vi "SVL Crest Factor (resampled) (1 Ch).vi"(6 "restart averaging (F)":bool, 8 "error in (no error)":errorcluster, 10 "even-angle channel info":T1={"channel name"="", "description"="", " channel info"={"sensor sensitivity"=1000.0, "engineering units"=1, "dB reference"=1.0, "custom label"="EU", "weighting filter"=0, "pregain"=0.0}} {"channel info"."pregain" format="%.2f"; "channel info"."weighting filter" items=["Linear", "A-weighting", "B-weighting", "C-weighting", "ITU-R 468-4", "Dolby", "CCITT", "C-message", "Wb", "Wc", "Wd", "We", "Wf", "Wh", "Wj", "Wk", "Wm", "AES17 20 kHz lowpass", "AES17 40 kHz lowpass", "AES17 20 kHz highpass", "AES17 40 kHz highpass"]; "channel info"."dB reference" format="%^.1e"; "channel info"."engineering units" items=["custom..."=0, "V"=1, "A"=21, "C"=30, "pC"=31, "s"=32, "-"=29, "Pa"=2, "N"=20, "g"=3, "m/s^2"=4, "m/s"=5, "m"=6, "mm/s"=12, "mm"=13, "micron/s"=14, "micron"=15, "in/s^2"=7, "in/s"=8, "in"=9, "mil/s"=10, "mil"=11, "rad/s^2"=16, "rad/s"=17, "rad"=18, "deg/s^2"=26, "deg/s"=27, "deg"=28, "RPM"=22, "cycle/s^2"=23, "Hz"=24, "cycle"=25, "strain"=19]; "channel info"."sensor sensitivity" format="%#_5f"}, 11 "even-angle signal [EU]":T5 {"even-angle signal" format="%.2f"; "dr" format="%.2f"; "r0" format="%.2f"}) -> (0 "error out":errorcluster, 1 "RMS level [EU rms]":dbl=nan format="%.2f", 2 "peak level [EU]":dbl=nan format="%.2f", 3 "crest factor":dbl=nan format="%.2f")   [LabVIEW 2017, in "SoundVib_VibrationLevel.lvlib"]
doc: "Computes the crest factor, peak level, and RMS level of <B>scaled signal [EU]</B> or <B>even-angle signal [EU]</B>. <B>scaled signal [EU]</B> should have a zero DC component. You can attenuate the DC component with hardware AC-coupling filters and with software high-pass filters. Wire data to the <B>scaled signal [EU]</B> input to determine the polymorphic instance to use or manually select the instance."
uses:
  <vilib>/addons/Sound and Vibration/svt_Level/SoundVib_VibrationLevel.lvlib
  <vilib>/addons/_NISVFA/_Shared subVIs/Controls/svc_Resampled Channel Info.ctl
  <vilib>/addons/_NISVFA/_Shared subVIs/Controls/svc_Channel Info.ctl
  <vilib>/addons/_NISVFA/_Shared subVIs/Controls/svc_Engineering Units Text Ring.ctl
  <vilib>/addons/_NISVFA/_Shared subVIs/Controls/svc_Weighting Filter Text Ring.ctl
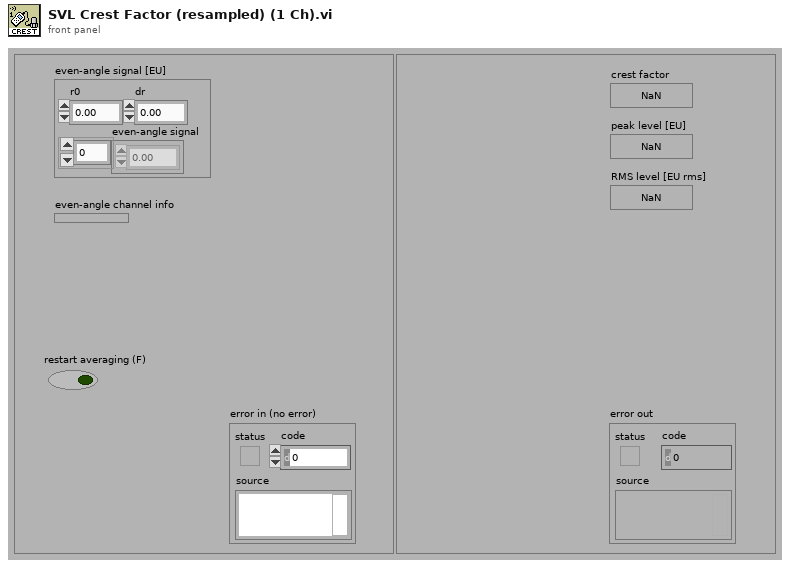
[diagram p1: front panel]
types:
  T1 = typedef "svc_Resampled Channel Info.ctl" = cluster{"channel name":string, "description":string, " channel info":T2}
  T2 = typedef "svc_Channel Info.ctl" = cluster{"sensor sensitivity":dbl, "engineering units":T3, "dB reference":dbl, "custom label":string, "weighting filter":T4, "pregain":dbl}
  T3 = typedef "svc_Engineering Units Text Ring.ctl" = u16
  T4 = typedef "svc_Weighting Filter Text Ring.ctl" = u16
  T5 = cluster{"r0":dbl, "dr":dbl, "even-angle signal":dbl[]}
  T6 = enum16{"RMS", "Running RMS", "Exp avg  ", "Dec exp avg ", "Peak", "Crest"}
  T7 = cluster{"r0":dbl, "dr":dbl, "even angle signal":dbl[]}
  T8 = enum16{"Reset filter", "Restart averaging", "Continue processing"}
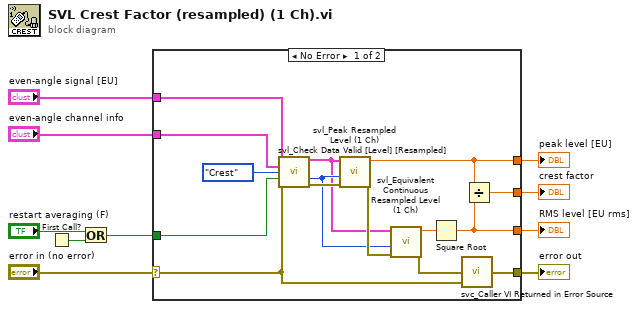
[diagram p0: block diagram]
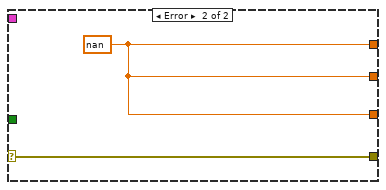
[diagram p2: hidden frame]
diagram:
  n1 = First Call?() -> (First Call?: T/F=w8:bool)
  n2 = Or(x="restart averaging (F)", y=w8) -> (x .or. y?=w7:bool)
  n3 = case shown="No Error" "error in (no error)" {
    tunnel: "even-angle signal [EU]" -> [w12 _]
    tunnel: [w15 w26] -> w5
    tunnel: [w22 w26] -> w4
    tunnel: [w21 w26] -> w3
    tunnel: [w20 w27] -> w2
    tunnel: w7 -> [w18 _]
    selector: "error in (no error)" -> [w11 w27]
    tunnel: "even-angle channel info" -> [w13 _]
    frame No Error {
      n4 = call <vilib>:"svl_Check Data Valid [Level] [Resampled].vi"("even angle signal"=w12, "even angle channel info"=w13, "Level Analysis"=T6."Crest", "restart averaging (F)"=w18, "error in (no error)"=w11) -> ("dup even angle signal"=w14:T7, "processing state"=w17:T8, "error out"=w19:errorcluster)  [unwired: 7 in, 1 out]
      n5 = call <vilib>:"svl_Peak Resampled Level (1 Ch).vi"("error in (no error)"=w19, "processing state"=w17, "even angle signal"=w14) -> ("error out"=w25:errorcluster, "peak level"=w15:dbl)  [unwired: 7 in]
      n6 = call <vilib>:"svl_Equivalent Continuous Resampled Level (1 Ch).vi"("error in (no error)"=w25, "processing state"=w17, "even angle signal"=w14) -> ("error out"=w24:errorcluster, "equivalent continuous level [EU^2 rms]"=w23:dbl)  [unwired: 7 in]
      n7 = Square Root(x=w23) -> (sqrt(x)=w21:dbl)
      n8 = call <vilib>:"svc_Caller VI Returned in Error Source.vi"("warning input to caller"=w11, "error in (no error)"=w24) -> ("error out"=w20:errorcluster)  [unwired: 3 in]
      n9 = Divide(x=w15, y=w21) -> (x/y=w22:dbl)
    }
    frame Error {
      w26 = nan
    }
  }
  "RMS level [EU rms]" <- w3
  "error out" <- w2
  "peak level [EU]" <- w5
  "crest factor" <- w4
